vi "2D_to_1D_Sum_sub.vi"(1 "2D array":ext[][](array[numeric])=[[-806.5101623390003, -4891.784794671002, -429.4833419949998, 1214.9466147229998, -1226.250826413, -47.48713166400046, -3205.3877712440008, 2910.7192305769995, 17.221259160999978, 732.7606715640002], [-806.5101623390003, -4891.784794671002, -429.4833419949998, 1214.9466147229998, -1226.250826413, -47.48713166400046, -3205.3877712440008, 2910.7192305769995, 17.221259160999978, 732.7606715640002], [-806.5101623390003, -4891.784794671002, -429.4833419949998, 1214.9466147229998, -1226.250826413, -47.48713166400046, -3205.3877712440008, 2910.7192305769995, 17.221259160999978, 732.7606715640002], [-806.5101623390003, -4891.784794671002, -429.4833419949998, 1214.9466147229998, -1226.250826413, -47.48713166400046, -3205.3877712440008, 2910.7192305769995, 17.221259160999978, 732.7606715640002]]) -> (0 "1D array":ext[](array[numeric]))   [LabVIEW 2021]
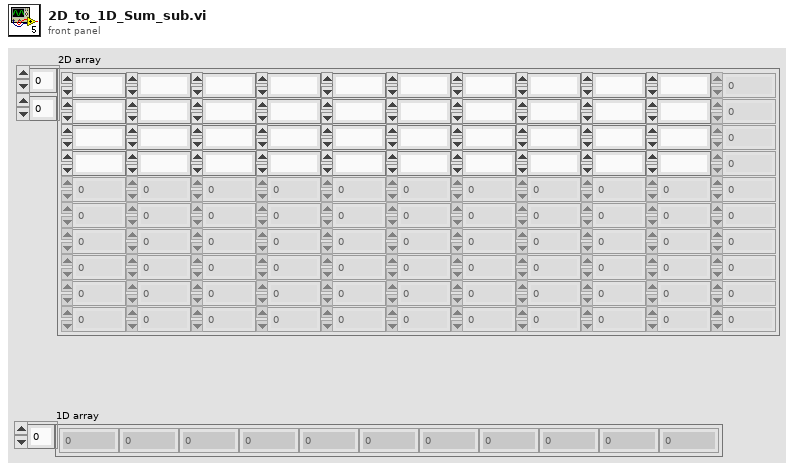
[diagram p1: front panel]
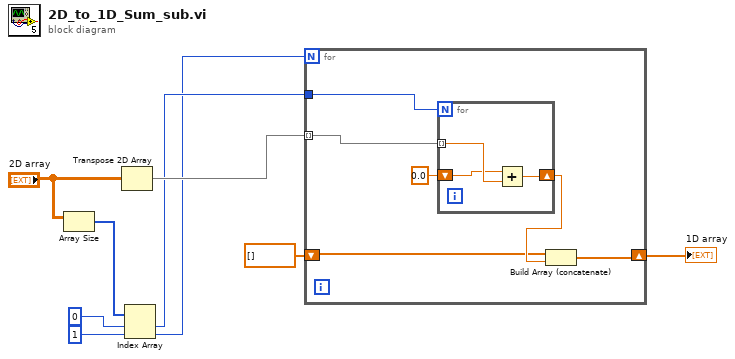
[diagram p0: block diagram]
diagram:
  n1 = Array Size(array="2D array") -> (size(s)=w5:i32[])
  n2 = Transpose 2D Array(2D array="2D array") -> (transposed array=w9:ext[][])
  n3 = Index Array(array=w5, index #1=0 ("인덱스"), index #2=1 ("인덱스")) -> (element #1=w2:i32, element #2=w1:i32)
  n4 = for {
    N: w1 -> [_]
    tunnel: w9 -> [w13] mode=indexing
    tunnel: w2 -> [w14]
    shift-right: [w12] -> w7
    shift-left: ext[] [] -> [w10]
    n5 = for {
      N: w14 -> [_]
      tunnel: w13 -> [w18] mode=indexing
      shift-right: [w17] -> w11
      shift-left: 0.0 -> [w16]
      n6 = Add(x=w16, y=w18) -> (x+y=w17:ext)
    }
    n7 = Build Array (concatenate)(w10, w11) -> (w12:ext[])
  }
  "1D array" <- w7
